vi "UHR-Fleezers Control (host) - 11.8.vi"() -> ()   [LabVIEW 2014] (continued)
        n2877 = Add(x=w4204, y=w4203) -> (x+y=w4202:dbl[][])
        n2878 = Divide(x=w4195, y=2) -> (x/y=w4193:dbl[][])
        n2879 = Divide(x=w4209, y=2) -> (x/y=w4154:dbl[][])
        n2880 = Divide(x=w4202, y=2) -> (x/y=w4156:dbl[][])
        n2881 = To Single Precision Float(number=w4189) -> (single precision float=w4188:sgl[][])
        n2882 = Transpose 2D Array(2D array=w4193) -> (transposed array=→"Data map":dbl[][])
        n2883 = To Single Precision Float(number=w4125) -> (single precision float=w4129:sgl[][])
        n2884 = To Single Precision Float(number=w4154) -> (single precision float=w4160:sgl[][])
        n2885 = To Single Precision Float(number=w4156) -> (single precision float=w4157:sgl[][])
        n2886 = call "IMAQ ArrayToImage"("Image Pixels (Float)"=w4188, "Image"=w4122) -> ("Image Out"=w4191:T2)  [unwired: 8 in, 1 out]
        n2887 = call "IMAQ ArrayToImage"("Image Pixels (Float)"=w4129, "Image"=w4121) -> ("Image Out"=w4131:T2)  [unwired: 8 in, 1 out]
        n2888 = call "IMAQ ArrayToImage"("Image Pixels (Float)"=w4160, "Image"=w4120) -> ("Image Out"=w4162:T2)  [unwired: 8 in, 1 out]
        n2889 = call "IMAQ ArrayToImage"("Image Pixels (Float)"=w4157, "Image"=w4119) -> ("Image Out"=w4159:T2)  [unwired: 8 in, 1 out]
        n2890 = call "IMAQ Symmetry"("Type of Symmetry"=w4190, "Image Src"=w4191) -> ("Image Dst Out"=w4186:T2)  [unwired: 3 in, 1 out]
        n2891 = call "IMAQ Symmetry"("Type of Symmetry"=w4130, "Image Src"=w4131) -> ("Image Dst Out"=w4127:T2)  [unwired: 3 in, 1 out]
        n2892 = call "IMAQ Symmetry"("Type of Symmetry"=w4161, "Image Src"=w4162) -> ("Image Dst Out"=→"Detection Laser X":T2)  [unwired: 3 in, 1 out]
        n2893 = call "IMAQ Symmetry"("Type of Symmetry"=w4158, "Image Src"=w4159) -> ("Image Dst Out"=→"Detection Laser Y":T2)  [unwired: 3 in, 1 out]
        n2894 = call "IMAQ Set Simple Calibration"("Calibration Axis Info"=T36 {"Origin Pixel"={"X"=0.0, "Y"=0.0}, "Angle Relative to Horizontal (deg)"=0.0, "Axis Reference"=0}, "Grid Descriptor"=T37 {"X Step"=0.3, "Y Step"=0.3, "Unit"=enum."Undefined"}, "Image"=w4186) -> ("Calibrated Image"=→"APD 1":T2)  [unwired: 7 in, 1 out]
        n2895 = call "IMAQ Set Simple Calibration"("Calibration Axis Info"=T36 {"Origin Pixel"={"X"=0.0, "Y"=0.0}, "Angle Relative to Horizontal (deg)"=0.0, "Axis Reference"=0}, "Grid Descriptor"=T37 {"X Step"=0.3, "Y Step"=0.3, "Unit"=enum."Undefined"}, "Image"=w4127) -> ("Calibrated Image"=→"APD 2":T2)  [unwired: 7 in, 1 out]
      }
    }
    n2896 = Subtract(x=w3570, y="APD 2 Offset") -> (x-y=w3567:waveform(dbl))
    n2897 = Subtract(x=w3572, y="APD 1 Offset") -> (x-y=w3568:waveform(dbl))
    n2898 = Index Array(array=w3587, index=3) -> (element=w3647:waveform(dbl))
    n2899 = Index Array(array=w3587, index=6) -> (element=w3644:waveform(dbl))
    n2900 = Build Array(w3568, w3567) -> (→"APD Chart":waveform(dbl)[])
    n2901 = Array Size(array=w3638) -> (size(s)=w3691:i32)
    n2902 = call <vilib>:"Std Deviation and Variance.vi"("X"=w3580) -> ("standard deviation"=w3579:dbl)  [unwired: 1 in, 2 out]
    n2903 = Add Array Elements(numeric array=w3580) -> (sum=w3582:u32)
    n2904 = Add Array Elements(numeric array=w3638) -> (sum=w3701:u32)
    n2905 = call <vilib>:"Std Deviation and Variance.vi"("X"=w3638) -> ("standard deviation"=w3637:dbl)  [unwired: 1 in, 2 out]
    n2906 = Divide(x="T1 offset_x (mV)", y=1000.0) -> (x/y=w3648:dbl)
    n2907 = Divide(x=w3579, y=w3578) -> (x/y=w3575:dbl)
    "Rate sigma (Hz) 2" <- w3575
    n2908 = Multiply(x=w3578, y=w3691) -> (x*y=w3581:dbl)
    "Int. Time (s)" <- w3581
    n2909 = Divide(x=w3582, y=w3581) -> (x/y=w3576:dbl)
    "APD 2 Rate (Hz)" <- w3576
    n2910 = Divide(x=w3701, y=w3581) -> (x/y=w3635:dbl)
    "APD 1 Rate (Hz)" <- w3635
    n2911 = Divide(x=w3637, y=w3578) -> (x/y=w3636:dbl)
    "Rate sigma (Hz)" <- w3636
    n2912 = Divide(x=w3575, y=w3576) -> (x/y=→"Sigma/Mean 2":dbl)
    n2913 = Divide(x=w3636, y=w3635) -> (x/y=→"s/Mean":dbl)
    n2914 = feedback-in #26("Calibration") -> ()
    n2915 = feedback #26(u16 1 ("Calibration")) -> (w3668:u16)
    n2916 = Divide(x="T2 offset_x (mV)", y=1000.0) -> (x/y=w3646:dbl)
    n2917 = case shown="0, Default" "Calibration" {
      tunnel: "T1 a_x (nm/V)" -> [_ w4085 w4106]
      tunnel: "T1 k_x (pN/nm)" -> [_ _ w4096]
      tunnel: "T2 a_x (nm/V)" -> [_ w4084 w4104]
      tunnel: "T2 k_x (pN/nm)" -> [_ _ w4097]
      tunnel: w3647 -> [w4067 w4082 w4102]
      tunnel: w3644 -> [w4066 w4080 w4100]
      tunnel: [w4067 w4079 w4099] -> w3677
      tunnel: [w4066 w4078 w4098] -> w3676
      tunnel: ["T1 X (V)" ("Label.Text") "T1 X (nm)" ("Label.Text") "T1 X (pN)" ("Label.Text")] -> w3665
      tunnel: ["T2 X (V)" ("Label.Text") "T2 X (nm)" ("Label.Text") "T2 X (pN)" ("Label.Text")] -> w3664
      tunnel: ["Position (V)" ("Label.Text") "Position (nm)" ("Label.Text") "Force (pN)" ("Label.Text")] -> w3666
      tunnel: w3646 -> [_ w4070 w4089]
      tunnel: w3648 -> [_ w4073 w4091]
      tunnel: ["Mean (V)" ("Label.Text") "Mean (nm)" ("Label.Text") "Mean (pN)" ("Label.Text")] -> w3661
      tunnel: ["Difference (V)" ("Label.Text") "Difference (nm)" ("Label.Text") "Difference (pN)" ("Label.Text")] -> w3595
      frame 0, Default {
      }
      frame 1 {
        n2918 = Unbundle By Name(w4082) -> ("Y"=w4086:dbl[])
        n2919 = Unbundle By Name(w4080) -> ("Y"=w4071:dbl[])
        n2920 = Subtract(x=w4086, y=w4073) -> (x-y=w4074:dbl[])
        n2921 = Subtract(x=w4071, y=w4070) -> (x-y=w4072:dbl[])
        n2922 = Multiply(x=w4072, y=w4084) -> (x*y=w4081:dbl[])
        n2923 = Multiply(x=w4085, y=w4074) -> (x*y=w4083:dbl[])
        n2924 = Bundle By Name(cluster=w4080, "Y"=w4081) -> (w4078:waveform(dbl))
        n2925 = Bundle By Name(cluster=w4082, "Y"=w4083) -> (w4079:waveform(dbl))
      }
      frame 2 {
        n2926 = Unbundle By Name(w4102) -> ("Y"=w4107:dbl[])
        n2927 = Unbundle By Name(w4100) -> ("Y"=w4105:dbl[])
        n2928 = Subtract(x=w4105, y=w4089) -> (x-y=w4090:dbl[])
        n2929 = Subtract(x=w4107, y=w4091) -> (x-y=w4092:dbl[])
        n2930 = Compound Arithmetic op=MULTIPLY(w4090, w4104, w4097) -> (w4101:dbl[])
        n2931 = Compound Arithmetic op=MULTIPLY(w4096, w4106, w4092) -> (w4103:dbl[])
        n2932 = Bundle By Name(cluster=w4100, "Y"=w4101) -> (w4098:waveform(dbl))
        n2933 = Bundle By Name(cluster=w4102, "Y"=w4103) -> (w4099:waveform(dbl))
      }
    }
    n2934 = Not Equal?(x=w3668, y="Calibration") -> (x != y?=w3625:bool)
    n2935 = case shown="True" w3625 {
      tunnel: w3666 -> [_ w4060]
      tunnel: w3665 -> [_ w4059]
      tunnel: w3664 -> [_ w4058]
      tunnel: w3661 -> [_ w4057]
      tunnel: w3595 -> [_ w4056]
      frame False {
      }
      frame True {
        n2936 = property on="Force" class="WFChart (strict)"("YScale.NameLbl.Text"=w4060) -> ()  [unwired: 2 in, 2 out]
        n2937 = property on="T2 X" class="DigNum (strict)"("Caption.Text"=w4058) -> ()  [unwired: 2 in, 2 out]
        n2938 = property on="T1 X" class="DigNum (strict)"("Caption.Text"=w4059) -> ()  [unwired: 2 in, 2 out]
        n2939 = property on="Mean" class="DigNum (strict)"("Caption.Text"=w4057) -> ()  [unwired: 2 in, 2 out]
        n2940 = property on="Difference" class="DigNum (strict)"("Caption.Text"=w4056) -> ()  [unwired: 2 in, 2 out]
      }
    }
    n2941 = Unbundle By Name(w3647) -> ("Y"=w3650:dbl[])
    n2942 = Unbundle By Name(w3644) -> ("Y"=w3653:dbl[])
    n2943 = Subtract(x=w3650, y=w3648) -> (x-y=w3651:dbl[])
    n2944 = Subtract(x=w3653, y=w3646) -> (x-y=w3652:dbl[])
    n2945 = Multiply(x=w3652, y="T2 a_x (nm/V)") -> (x*y=w3440:dbl[])
    n2946 = Multiply(x="T1 a_x (nm/V)", y=w3651) -> (x*y=w3441:dbl[])
    n2947 = Not(x="Trap Trig. Fl.") -> (.not. x?=w3477:bool)
    n2948 = Multiply(x=w3676, y=-1.0) -> (x*y=w3655:waveform(dbl))
    n2949 = Subtract(x=w3441, y=w3440) -> (x-y=w3643:dbl[])
    n2950 = Unbundle By Name(w3676) -> ("Y"=w3614:dbl[])
    n2951 = Unbundle By Name(w3677) -> ("Y"=w3442:dbl[])
    n2952 = Negate(x=w3643) -> (-x=w3438:dbl[])
    n2953 = Build Array(w3677, w3655) -> (→"Force":waveform(dbl)[])
    n2954 = Subtract(x=w3438, y="Offset (nm)") -> (x-y=w3612:dbl[])
    n2955 = case shown="True" "Read Lateness and Rel Phase" {
      tunnel: w3458 -> [w4033 w4055]
      tunnel: w3457 -> [w4034 w4054]
      tunnel: [w4033 w4053] -> w3641
      tunnel: [w4034 w4052] -> w3640
      frame False {
      }
      frame True {
        n2956 = xnode "Read/Write Control"("FPGA VI Reference In"=w4055, "error in"=w4054) -> ("FPGA VI Reference Out"=w4053:T19, "error out"=w4052:errorcluster, "GI Relative phase"=→"GI relative phase":i16, "Relative phase"=→"Relative phase (AI1)":i16, "AI Late Counter"=→"Late Counter (AI1)":u8, "GI Late Counter"=→"GI Late Counter":u8, "MCL Late Counter"=→"MCL Late Counter":u8, "MCL Relative Phase"=→"Relative Phase (MCL)":i16, "APD Acq Relative Phase"=→"APD Acq Relative Phase":i16, "APD 1 Gate Relative Phase"=→"APD 1 Gate Relative Phase":i16, "APD 2 Gate Relative Phase"=→"APD 2 Gate Relative Phase":i16, "APD Acq Late Counter"=→"APD Acq Late Counter":u8, "APD 1 Gate Late Counter"=→"APD 1 Gate Late Counter":u8, "APD 2 Gate Late Counter"=→"APD 2 Gate Late Counter":u8, "Green FB Relative Phase"=→"Relative phase (Green FB)":i16, "GI Relative phase 2"=→"GI relative phase 2":i16, "GI Late Counter 2"=→"GI Late Counter 2":u8, "Trap Pos FIFO Timeout"=→"Trap Pos FIFO Timeout":u16, "Trap AI FIFO Timeout"=→"Trap AI FIFO Timeout":u16)
      }
    }
    n2957 = call-poly <vilib>:"Mean.vi"("X"=w3614) -> ("mean"=w3444:dbl)  [unwired: 1 out]
    "T2 X" <- w3444
    n2958 = Negate(x=w3614) -> (-x=w3615:dbl[])
    n2959 = call-poly <vilib>:"Mean.vi"("X"=w3442) -> ("mean"=w3445:dbl)  [unwired: 1 out]
    "T1 X" <- w3445
    n2960 = Negate(x=w3444) -> (-x=w3443:dbl)
    n2961 = Bundle By Name(cluster=w3647, "Y"=w3612) -> (w3586:waveform(dbl))
    "Bead Separation" <- w3586
    n2962 = Add(x=w3442, y=w3615) -> (x+y=w3616:dbl[])
    n2963 = Add(x=w3445, y=w3443) -> (x+y=w3663:dbl)
    n2964 = Subtract(x=w3445, y=w3443) -> (x-y=→"Difference":dbl)
    n2965 = Divide(x=w3616, y=2.0) -> (x/y=→"Vec Mean of T1 T2":dbl[])
    n2966 = Divide(x=w3663, y=2.0) -> (x/y=w3618:dbl)
    "Mean" <- w3618
    n2967 = feedback-in #27("Trap Trig. Fl.") -> ()
    n2968 = feedback #27("Trap Trig. Fl.") -> (w3475:bool)
    n2969 = And(x=w3477, y=w3475) -> (x .and. y?=w3476:bool)
    n2970 = case "If have just turned off triggering" shown="True" w3476 {
      tunnel: w3458 -> [_ w3863]
      tunnel: w3457 -> [_ w3862]
      frame False {
      }
      frame True {
        w3861 = FALSE ("FPGA Trap Trig")
        n2971 = xnode "Read/Write Control"("FPGA VI Reference In"=w3863, "error in"=w3862, "FPGA Trap Trig"=w3861) -> ("FPGA VI Reference Out"=w3860:T19, "error out"=w3859:errorcluster)
        n2972 = xnode "Read/Write Control"("FPGA VI Reference In"=w3860, "error in"=w3859, "TTrig?"=w3861) -> ()  [unwired: 2 out]
        n2973 = local write "Initializing"(FALSE ("Initializing")) -> ()
        n2974 = local write "Triggered"(FALSE ("Triggered")) -> ()
        n2975 = local write "Waiting"(FALSE ("Waiting")) -> ()
      }
    }
    n2976 = Not(x=w3475) -> (.not. x?=w3488:bool)
    n2977 = And(x="Trap Trig. Fl.", y=w3488) -> (x .and. y?=w3485:bool)
    n2978 = local read "Tether"() -> (w3619:bool)
    n2979 = Or(x=w3485, y="Reinitialize") -> (x .or. y?=w3471:bool)
    n2980 = feedback #28(w3481) -> (w3486:string)
    n2981 = Select(t=w3481, s=w3485, f=w3486) -> (s? t:f=w3480:string)
    n2982 = Select(t=w3481, s="Reinitialize", f=w3480) -> (s? t:f=w3479:string)
    n2983 = feedback #29(0) -> (w3483:i32)
    n2984 = feedback #30(w3612) -> (w3611:dbl[])
    n2985 = Build Array (concatenate)(w3612, w3611) -> (w3439:dbl[])
    n2986 = case "For determining if there is a tether still" shown="True" w3619 {
      tunnel: w3618 -> [_ w3987]
      frame False {
      }
      frame True {
        n2987 = Greater?(x="Lost Tether Alarm Threshold (pN)", y=w3987) -> (0:w3985:bool)
        n2988 = case shown="True" w3985 {
          frame False {
          }
          frame True {
            w3988 = TRUE
            w3992 = FALSE ("Multiple tether")
            w3993 = FALSE ("Value (Signaling)")
            n2989 = flat-sequence {
              frame #0 {
                # "stop only if saving"
                n2990 = local read "Saving..."() -> (w4005:bool)
                n2991 = And(x=w4005, y="TA Cancel Save?") -> (x .and. y?=w4004:bool)
                n2992 = local write "Stop Saving"(w4004) -> ()
              }
              frame #1 {
                n2993 = case shown="True" "TA Green Off?" {
                  frame False {
                  }
                  frame True {
                    w4008 = FALSE ("Fl. Triggered...")
                    n2994 = local write "Fl. Triggered..."(w4008) -> ()
                    n2995 = property on="Green Laser ON/Interlacing" class="Bool (strict)"("Val(Sgnl)"=w4008) -> ()  [unwired: 2 in, 2 out]
                  }
                }
              }
            }
            n2996 = local read "Time tether formed"() -> (w3999:timestamp)
            n2997 = Get Date/Time In Seconds() -> (seconds since 1Jan1904=w4000:timestamp)
            n2998 = Subtract(x=w4000, y=w3999) -> (x-y=w3998:dbl)
            n2999 = Number To Decimal String(number=w3998) -> (decimal integer string=w3995:string)  [unwired: 1 out]
            n3000 = local read "Messages"() -> (w4002:string)
            n3001 = call <vilib>:"Beep.vi"("use system alert? (T)"=FALSE, "duration (msec)"=u32 200, "frequency (Hz)"=u32 200) -> ()  [unwired: 9 out]
            n3002 = Concatenate Strings("Lost tether (" ("Message to add"), w3995, " s)." ("string")) -> (w3997:string)
            n3003 = local write "Tether"(FALSE ("Tether")) -> ()
            n3004 = call "Update messages.vi"("Message to add"=w3997, "Old message string"=w4002) -> ("New message string"=w4001:string)
            n3005 = local write "Messages"(w4001) -> ()
            n3006 = local write "Pause dwell"(w3993) -> ()
            n3007 = property on="Fl. Triggered..." class="Bool (strict)"("Val(Sgnl)"=w3993) -> ()  [unwired: 2 in, 2 out]
            n3008 = local write "Dip for Protein"(w3993) -> ()
            n3009 = property on="Trap Pos. FB ON" class="Bool (strict)"("Val(Sgnl)"=w3993) -> ()  [unwired: 2 in, 2 out]
            n3010 = property on="Trap Trig. Fl." class="Bool (strict)"("Val(Sgnl)"=w3993) -> ()  [unwired: 2 in, 2 out]
            n3011 = local write "Multiple tether"(w3992) -> ()
            n3012 = local write "Bad fit"(w3992) -> ()
            n3013 = local write "Hysteresis"(w3992) -> ()
            n3014 = local write "Good tether"(w3992) -> ()
            n3015 = local write "Save scans"(w3988) -> ()
            n3016 = local write "Restart DMA? (AOD)"(w3988) -> ()
          }
        }
      }
    }
    n3017 = case "For triggering actions based on the trap position (e.g., turning the excitation laser on if trap under feedback moves so far)" shown="True" "Trap Trig. Fl." {
      tunnel: w3466 -> [_ w3876]
      tunnel: w3479 -> [_ w3875]
      tunnel: ["" ("t") w3874] -> w3487
      tunnel: w3471 -> [_ w3873]
      tunnel: [0 ("t") w3872] -> w3484
      tunnel: w3483 -> [_ w3871]
      tunnel: w3458 -> [_ w3870]
      tunnel: w3457 -> [_ w3869]
      frame False {
      }
      frame True {
        n3018 = case shown="\"Wait for trigger\"" w3875 {
          tunnel: w3876 -> [w3893 _ _ w3941]
          tunnel: [w3890 w3922 "" ("t") w3944] -> w3874
          tunnel: w3873 -> [_ _ _ w3932]
          tunnel: [w3889 w3919 0 ("t") w3933] -> w3872
          tunnel: w3871 -> [_ w3921 _ w3939]
          tunnel: w3870 -> [w3878 w3916 _ w3935]
          tunnel: w3869 -> [w3877 w3915 _ w3934]
          frame "Wait for trigger" {
            n3019 = local read "Trap Trig. (FPGA)"() -> (w3881:bool)
            n3020 = Subtract(x=w3893, y="Mean T1 Position\nto compare (nm)") -> (x-y=w3886:dbl[])
            n3021 = call <vilib>:"Std Deviation and Variance.vi"("X"=w3886) -> ("mean"=→"mean":dbl, "standard deviation"=→"standard\ndeviation":dbl)  [unwired: 1 in, 1 out]
            n3022 = Array Max & Min(array=w3886) -> (max value=→"max value":dbl, min value=→"min value":dbl)  [unwired: 2 out]
            n3023 = Greater?(x=w3886, y="Threshold (nm)") -> (0:w3896:bool[])
            n3024 = case shown="True" w3881 {
              tunnel: w3878 -> [_ w3902]
              tunnel: w3877 -> [_ w3901]
              tunnel: [FALSE ("TTrig?") w3900] -> w3884
              frame False {
              }
              frame True {
                n3025 = xnode "Read/Write Control"("FPGA VI Reference In"=w3902, "error in"=w3901) -> ("TTrig?"=w3900:bool)  [unwired: 2 out]
              }
            }
            n3026 = Or Array Elements(Boolean array=w3896) -> (logical OR=w3883:bool)
            n3027 = Select(t=w3884, s=w3881, f=w3883) -> (s? t:f=w3882:bool)
            n3028 = Not(x=w3881) -> (.not. x?=w3880:bool)
            n3029 = And(x=w3882, y=w3880) -> (x .and. y?=w3879:bool)
            n3030 = Select(t="Triggered", s=w3882, f="Wait for trigger") -> (s? t:f=w3890:string)
            n3031 = case shown="True" w3882 {
              tunnel: [0 0] -> w3889
              tunnel: w3878 -> [_ w3907]
              tunnel: w3877 -> [_ w3906]
              frame False {
                "Waiting" <- TRUE ("Waiting")
              }
              frame True {
                n3032 = xnode "Read/Write Control"("FPGA VI Reference In"=w3907, "error in"=w3906, "TTrig?"=FALSE) -> ()  [unwired: 2 out]
                n3033 = local read "Messages"() -> (w3910:string)
                n3034 = call <vilib>:"Beep.vi"() -> ()  [unwired: 12 in]
                n3035 = call "Update messages.vi"("Message to add"="Unwinding trigger.", "Old message string"=w3910) -> ("New message string"=w3911:string)
                n3036 = local write "Messages"(w3911) -> ()
                n3037 = local write "Waiting"(FALSE ("Waiting")) -> ()
                "Triggered" <- TRUE ("Triggered")
              }
            }
            n3038 = case "Only need to turn on laser if host triggered" shown="True" w3879 {
              frame False {
              }
              frame True {
                n3039 = property on="Green Laser ON/Interlacing" class="Bool (strict)"("Val(Sgnl)"=TRUE ("Value (Signaling)")) -> ()  [unwired: 2 in, 2 out]
              }
            }
          }
          frame "Triggered" {
            n3040 = local read "Trap Trig. (FPGA)"() -> (w3918:bool)
            n3041 = Increment(x=w3921) -> (x+1=w3919:i32)
            n3042 = Greater Or Equal?(x=w3919, y="Fl. ON time (n)") -> (x >= y?=w3917:bool)
            n3043 = Select(t="Wait for trigger", s=w3917, f="Triggered" ("t")) -> (s? t:f=w3922:string)
            n3044 = And(x=w3917, y=w3918) -> (x .and. y?=w3914:bool)
            n3045 = case shown="True" w3914 {
              tunnel: w3916 -> [_ w3926]
              tunnel: w3915 -> [_ w3925]
              frame False {
              }
              frame True {
                n3046 = xnode "Read/Write Control"("FPGA VI Reference In"=w3926, "error in"=w3925, "FPGA Trap Trig"=TRUE) -> ()  [unwired: 2 out]
              }
            }
            n3047 = case shown="True" w3917 {
              frame False {
              }
              frame True {
                w3928 = FALSE ("Value (Signaling)")
                n3048 = local write "Triggered"(w3928) -> ()
                n3049 = local write "Waiting"(TRUE ("Waiting")) -> ()
                n3050 = property on="Green Laser ON/Interlacing" class="Bool (strict)"("Val(Sgnl)"=w3928) -> ()  [unwired: 2 in, 2 out]
              }
            }
          }
          frame "Do nothing" {
          }
          frame "Initialize", Default {
            n3051 = Increment(x=w3939) -> (x+1=w3943:i32)
            n3052 = Select(t=1, s=w3932, f=w3943) -> (s? t:f=w3933:i32)
            n3053 = feedback #31(w3941) -> (w3947:dbl[])
            n3054 = Build Array (concatenate)(w3941, w3947) -> (w3940:dbl[])
            n3055 = Greater Or Equal?(x=w3933, y="Wait to get offset (n)") -> (x >= y?=w3936:bool)
            n3056 = Select(t=w3941, s=w3932, f=w3940) -> (s? t:f=w3942:dbl[])
            n3057 = feedback-in #31(w3942) -> ()
            n3058 = call-poly <vilib>:"Mean.vi"("X"=w3942) -> ("mean"=w3937:dbl)  [unwired: 1 out]
            n3059 = local write "Mean T1 Position\nto compare (nm)"(w3937) -> ()
            n3060 = case shown="True" w3932 {
              tunnel: w3935 -> [_ w3953]
              tunnel: w3934 -> [_ w3952]
              frame False {
              }
              frame True {
                w3949 = FALSE ("FPGA Trap Trig")
                n3061 = xnode "Read/Write Control"("FPGA VI Reference In"=w3953, "error in"=w3952, "FPGA Trap Trig"=w3949) -> ("FPGA VI Reference Out"=w3951:T19, "error out"=w3950:errorcluster)
                n3062 = xnode "Read/Write Control"("FPGA VI Reference In"=w3951, "error in"=w3950, "TTrig?"=w3949) -> ()  [unwired: 2 out]
              }
            }
            n3063 = Select(t="Wait for trigger", s=w3936, f="Initialize") -> (s? t:f=w3944:string)
            n3064 = case shown="True" w3936 {
              tunnel: w3937 -> [_ w3956]
              tunnel: w3935 -> [_ w3965]
              tunnel: w3934 -> [_ w3964]
              frame False {
                n3065 = local write "Waiting"(FALSE ("Waiting")) -> ()
                "Initializing" <- TRUE ("Initializing")
              }
              frame True {
                n3066 = local read "Threshold (nm)"() -> (w3968:dbl)
                n3067 = local read "AOM X Cal (nm/MHz)"() -> (w3967:dbl)
                n3068 = Add(x=w3956, y=w3968) -> (x+y=w3969:dbl)
                n3069 = Divide(x=w3969, y=w3967) -> (x/y=w3966:dbl)
                n3070 = call "IR AOM freq to word.vi"("Frequency In (MHz)"=w3966) -> ("Frequency Word Out (double)"=w3963:dbl)
                n3071 = local write "Initializing"(FALSE ("Initializing")) -> ()
                n3072 = local write "Waiting"(TRUE ("Waiting")) -> ()
                n3073 = To Quad Integer(1:w3963) -> (0:w3962:i64)
                n3074 = xnode "Read/Write Control"("FPGA VI Reference In"=w3965, "error in"=w3964, "FPGA TTrig Thresh"=w3962) -> ("FPGA VI Reference Out"=w3959:T19, "error out"=w3958:errorcluster)
                n3075 = xnode "Read/Write Control"("FPGA VI Reference In"=w3959, "error in"=w3958, "FPGA Trap Trig"=TRUE) -> ()  [unwired: 2 out]
              }
            }
          }
        }
      }
    }
    n3076 = feedback-in #28(w3487) -> ()
    n3077 = feedback-in #29(w3484) -> ()
    n3078 = Split 1D Array(array=w3439, index=w3501) -> (first subarray=w3608:dbl[])  [unwired: 1 out]
    n3079 = feedback-in #30(w3608) -> ()
    n3080 = call-poly <vilib>:"Mean.vi"("X"=w3608) -> ("mean"=w3607:dbl)  [unwired: 1 out]
    "Bead Mean (nm)" <- w3607
    n3081 = Subtract(x=w3608, y=w3607) -> (x-y=w3606:dbl[])
    n3082 = Square(x=w3606) -> (x^2=w3605:dbl[])
    n3083 = call-poly <vilib>:"Mean.vi"("X"=w3605) -> ("mean"=w3604:dbl)  [unwired: 1 out]
    n3084 = Square Root(x=w3604) -> (sqrt(x)=w3603:dbl)
    n3085 = Multiply(x=10.0, y=w3603) -> (x*y=→"RMS (Å)":dbl)
    n3086 = xnode ("Read/Write Control")("FPGA VI Reference In"=w3641, "error in"=w3640) -> ("FPGA VI Reference Out"=w3469:T19, "error out"=w3468:errorcluster, "AI2 Y Sum Set 1"=w3746:i16, "AI2 Y Sum Set 2"=w3745:i16, "AI1 X Set 1"=w3532:fxp<+/-,16,1>, "AI1 X Set 2"=w3531:fxp<+/-,16,1>, "Trap Pos FB Int Signal"=→"Trap Pos FB Int Signal":fxp<+/-,24,9>, "Trap Pos FB Int-Norm Signal"=→"Trap Pos FB Int-Norm Signal":fxp<+/-,16,1>, "Trap Pos FB Action"=w3525:i64, "Scanning"=→"AOD Scanning":bool, "Scan I"=→"AOD Scan I":u64, "Scanning MCL"=w3748:bool, "Scan I (MCL)"=→"MCL Scan I":u64, "Green FB Signals"=w3686:T47, "Trap Pos FB Action"=w3456:i64, "Wiggling 1"=→"Wiggling T1":bool, "TTrig Fin Thresh"=w3452:i64, "Wiggling 2"=→"Wiggling T2":bool)  [unwired: 2 out]
    "MCL Scanning" <- w3748
    "Trap Pos FB Action" <- w3525
    n3087 = local read "FB Trig Integrate"() -> (w3450:u32)
    n3088 = Divide(x=w3456, y=w3450) -> (x/y=w3449:dbl)
    "TTrig Sig (Int)" <- w3449
    n3089 = Divide(x=w3452, y=w3450) -> (x/y=w3447:dbl)
    "TTrig Fin Thresh (Int)" <- w3447
    n3090 = local read "AOM X Cal (nm/MHz)"() -> (w3455:dbl)
    n3091 = local read "AI2 (V)"() -> (w3747:cluster{"Set 1":dbl, "Set 2":dbl})
    n3092 = Bundle By Name(cluster=w3747, "Set 1"=w3746, "Set 2"=w3745) -> (w3743:cluster{"Set 1":dbl, "Set 2":dbl})
    n3093 = Divide(x=w3525, y=327.67) -> (x/y=w3434:dbl)
    n3094 = local read "Trap X (AI1)"() -> (w3545:T10)
    n3095 = call "IR AOM word double to freq.vi"("Frequency Word In (double)"=w3447) -> ("Frequency Out (MHz)"=w3446:dbl)
    n3096 = call "IR AOM word double to freq.vi"("Frequency Word In (double)"=w3449) -> ("Frequency Out (MHz)"=w3448:dbl)
    n3097 = Divide(x=w3743, y=3276.7) -> (x/y=w3742:cluster{"Set 1":dbl, "Set 2":dbl})
    n3098 = Multiply(x=w3448, y=w3455) -> (x*y=w3454:dbl)
    "TTrig Sig (nm)" <- w3454
    n3099 = Multiply(x=w3446, y=w3455) -> (x*y=w3453:dbl)
    "TTrig Fin Thresh (nm)" <- w3453
    n3100 = local write "AI2 (V)"(w3742) -> ()
    n3101 = local read "Trap Pos. FB Range"() -> (w3433:T12)
    n3102 = Bundle(cluster=w3545, "Trap 1"=w3532, "Trap 2"=w3531) -> (→"Trap X (AI1)":T10)
    n3103 = Bundle(w3454, w3453) -> (→"TTrig":cluster{dbl, dbl})  [unwired: 1 in]
    n3104 = Unbundle(w3433) -> ("output high"=w3432:fxp<+/-,64,32>)  [unwired: 1 out]
    n3105 = Divide(x=w3434, y=w3432) -> (x/y=→"Action (%)":dbl)
    n3106 = Divide(x=w3686, y=3276.7) -> (x/y=w3682:T48)
    n3107 = Unbundle By Name(w3682) -> ("Green FB Ch 0"=w3685:dbl, "Green FB Ch 1"=w3684:dbl, "Green FB Ch 2"=w3683:dbl)
    n3108 = Divide(x=w3685, y=w3683) -> (x/y=w3681:dbl)
    n3109 = Divide(x=w3684, y=w3683) -> (x/y=w3680:dbl)
    n3110 = flat-sequence "To save data" {
      tunnel: [w4829] -> w3766
      tunnel: [w4830] -> w3765
      tunnel: w3717 -> [w4802]
      tunnel: w3474 -> [w4827]
      tunnel: ["Save Calibration"] -> w3739
      tunnel: w3736 -> [w4826]
      tunnel: [w4820] -> w3735
      tunnel: [w4817] -> w3734
      tunnel: [w4814] -> w3733
      tunnel: w3716 -> [w4816]
      tunnel: w3623 -> [w4810]
      tunnel: [w4810] -> w3622
      tunnel: ["Start Saving"] -> w3588
      tunnel: [w4804] -> w3514
      tunnel: [w4803] -> w3513
      tunnel: w3766 -> [w5069]
      tunnel: w3765 -> [w5068]
      tunnel: w3515 -> [w5067]
      tunnel: w3739 -> [w5066]
      tunnel: w3735 -> [w5064]
      tunnel: w3734 -> [w5063]
      tunnel: w3733 -> [w5062]
      tunnel: w3597 -> [w5061]
      tunnel: w3633 -> [w5060]
      tunnel: w3622 -> [w5059]
      tunnel: w3588 -> [w5058]
      tunnel: w3586 -> [w5057]
      tunnel: w3562 -> [w5056]
      tunnel: w3514 -> [w5055]
      tunnel: w3513 -> [w5054]
      tunnel: w3512 -> [w5053]
      tunnel: w3435 -> [w5052]
      frame #0 {
        n3111 = Or(x="Save N Sets", y="Start Saving") -> (x .or. y?=w4811:bool)
        n3112 = To Double Precision Float(number=w4826) -> (double precision float=w4821:dbl)
        n3113 = Build Array(w4811, "Save Calibration", w4802, w4816) -> (w4825:bool[])
        n3114 = Compound Arithmetic op=OR("Save Calibration", w4802, w4811, w4816) -> (w4828:bool)
        n3115 = Boolean Array To Number(Boolean array=w4825) -> (number=w4823:u32)
        n3116 = feedback #32(FALSE ("Save APD Data\nwith Trap Data")) -> (w4805:bool)
        n3117 = feedback #33(refnum<k0> refnum) -> (w4831:refnum<file>)
        n3118 = feedback #34(refnum<k0> refnum) -> (w4807:refnum<file>)
        n3119 = feedback #35(FALSE ("Save APD Data\nwith Trap Data")) -> (w4815:bool)
        n3120 = feedback #36(refnum<k0> refnum) -> (w4818:refnum<file>)
        n3121 = feedback #37(0) -> (w4833:i32)
        n3122 = feedback #38() -> (w4822:u32)  [unwired: 1 out]
        n3123 = case shown="True" w4828 {
          tunnel: [w4840 1] -> w4829
          tunnel: w4833 -> [w4842 _]
          tunnel: [w4841 w4860] -> w4830
          tunnel: w4831 -> [w4841 _]
          tunnel: w4827 -> [_ w4880]
          tunnel: w4821 -> [_ w4878]
          tunnel: w4823 -> [_ w4881]
          tunnel: [w4839 w4859] -> w4820
          tunnel: w4822 -> [w4839 _]
          tunnel: [w4838 w4857] -> w4817
          tunnel: w4818 -> [w4838 _]
          tunnel: [w4837 w4856] -> w4814
          tunnel: w4815 -> [w4837 _]
          tunnel: "Start Saving" -> [_ w4854]
          tunnel: w4810 -> [_ w4853]
          tunnel: [w4836 w4844] -> w4803
          tunnel: w4807 -> [w4836 _]
          tunnel: [w4835 w4843] -> w4804
          tunnel: w4805 -> [w4835 _]
          frame False {
            n3124 = Increment(x=w4842) -> (x+1=w4840:i32)
          }
          frame True {
            w4850 = FALSE ("Start Saving")
            w4855 = 9.0  # File Version
            w4863 = FALSE ("prepend array or string size? (T)")
            w4861 = T24."big-endian, network order" ("byte order (0:big-endian, network order)")
            n3125 = local read "BD 1 Frequency 1 (MHz)"() -> (w4877:dbl)
            n3126 = local read "BD 2 Frequency 1 (MHz)"() -> (w4876:dbl)
            n3127 = local read "BD 1 Frequency 2 (MHz)"() -> (w4875:dbl)
            n3128 = local read "BD 2 Frequency 2 (MHz)"() -> (w4874:dbl)
            n3129 = local read "BD 1 Frequency 3 (MHz)"() -> (w4873:dbl)
            n3130 = local read "BD 2 Frequency 3 (MHz)"() -> (w4872:dbl)
            n3131 = Array Size(array=w4853) -> (size(s)=w4852:i32)
            n3132 = To Double Precision Float(number=w4852) -> (double precision float=w4851:dbl)
            n3133 = local write "Save Calibration"(w4850) -> ()
            n3134 = local write "Start Saving"(w4850) -> ()
            n3135 = Build Array("Save APD Data\nwith Trap Data", "Save Trap Pos. Data") -> (w4847:bool[])
            n3136 = Boolean Array To Number(Boolean array=w4847) -> (number=w4846:u32)
            n3137 = Build Array(w4877, w4876, w4875, w4874, w4873, w4872) -> (w4871:dbl[])
            n3138 = case shown="1, Default" w4881 {
              tunnel: w4880 -> [w4954 w4976 w4992 w5030]
              tunnel: w4851 -> [w4959 w4983 w5012 w5049]
              tunnel: w4878 -> [w4958 w4982 w5011 w5048]
              tunnel: [w4955 w4978 w5003 w5040] -> w4869
              tunnel: [w4947 "Cal sets to save" w4993 w5031] -> w4859
              tunnel: w4871 -> [w4956 w4979 w5005 w5042]
              tunnel: "Save APD Data\nwith Trap Data" -> [w4953 _ w4989 w5028]
              tunnel: [w4953 FALSE ("Save APD Data\nwith Trap Data") w4989 w5028] -> w4856
              tunnel: w4855 -> [w4950 w4973 w4987 w5026]
              tunnel: w4854 -> [w4949 _ _ _]
              tunnel: [w4941 "Active cal?" w4986 w5016] -> w4843
              tunnel: "Save Trap Pos. Data" -> [w4941 _ w4986 w5016]
              tunnel: w4846 -> [w4940 _ w4985 w5015]
              frame 1, Default {
                # "timeseries"
                n3139 = case shown="True" "Profile" {
                  tunnel: [w4962 w4966] -> w4945
                  tunnel: [w4962 w4965] -> w4944
                  tunnel: [w4962 w4964] -> w4943
                  tunnel: [w4962 w4963] -> w4942
                  frame False {
                    w4962 = 0.0 ("f")
                  }
                  frame True {
                    n3140 = local read "Current Position"() -> (w4967:cluster{dbl, dbl, dbl})
                    n3141 = local read "Y change (mm)"() -> (w4963:dbl)
                    n3142 = Unbundle(w4967) -> (w4966:dbl, w4965:dbl, w4964:dbl)
                  }
                }
                n3143 = local read "Save ave N"() -> (w4961:dbl)
                n3144 = Multiply(x=w4961, y=w4954) -> (x*y=w4960:dbl)
                n3145 = To Double Precision Float(number=w4940) -> (double precision float=w4952:dbl)
                n3146 = Select(t=4.0, s="Profile", f=0.0) -> (s? t:f=w4936:dbl)
                n3147 = Build Array(w4950, w4954, w4960, w4959, w4958, w4936) -> (w4957:dbl[])
                n3148 = Build Array(w4952, w4945, w4944, w4943, w4942) -> (w4951:dbl[])
                n3149 = Select(t=u32 4000000000, s=w4949, f="N sets to save") -> (s? t:f=w4947:u32)
                n3150 = Build Array (concatenate)(w4957, w4956, w4951) -> (w4955:dbl[])
              }
              frame 2 {
                w4975 = 0.0 ("f")
                # "If doing active calibration,\nalso save trap position file"
                # "calibration"
                n3151 = property on="Wiggle" class="Bool (strict)"("Val(Sgnl)"="Active cal?") -> ()  [unwired: 2 in, 2 out]
                n3152 = Select(t=2.0, s="Active cal?", f=0.0) -> (s? t:f=w4969:dbl)
                n3153 = Build Array(w4969, w4975, w4975, w4975, w4975) -> (w4974:dbl[])
                n3154 = Build Array(w4973, w4976, w4976, w4983, w4982, 1.0 ("t")) -> (w4980:dbl[])
                n3155 = Build Array (concatenate)(w4980, w4979, w4974) -> (w4978:dbl[])
                "Calibrating..." <- TRUE ("Calibrating...")
              }
              frame 4 {
                w4990 = 0.0 ("f")
                # "scan dir (x/y = 0/1)"
                # "cycles/step"
                # "n scans (f/b)"
                # "steps"
                # "freq. range"
                # "AOD raster scan"
                n3156 = local read "Number of F/B Scans (AOD)"() -> (w4997:u16)
                n3157 = local read "Cycles/step (AOD)"() -> (w4999:u64)
                n3158 = local read "Scan Range (MHz)"() -> (w5002:dbl)
                n3159 = local read "Scan steps (AOD)"() -> (w5001:u64)
                n3160 = local read "Scan BD"() -> (w5009:bool)
                n3161 = local read "Save ave N"() -> (w5014:dbl)
                n3162 = Boolean To (0,1)(Boolean=w5009) -> (0, 1=w5008:i16)
                n3163 = To Double Precision Float(number=w4997) -> (double precision float=w4996:dbl)
                n3164 = To Double Precision Float(number=w5001) -> (double precision float=w5000:dbl)
                n3165 = To Double Precision Float(number=w4999) -> (double precision float=w4998:dbl)
                n3166 = To Double Precision Float(number=w5008) -> (double precision float=w5007:dbl)
                n3167 = Multiply(x=w5014, y=w4992) -> (x*y=w5013:dbl)
                n3168 = To Double Precision Float(number=w4985) -> (double precision float=w4991:dbl)
                n3169 = Build Array(w4991, w4990, w4990, w4990, w4990) -> (w4988:dbl[])
                n3170 = local read "N sets should be saved"() -> (w4994:dbl)
                n3171 = Build Array(w5007, w5002, w5000, w4998, w4996) -> (w5004:dbl[])
                n3172 = Build Array(w4987, w4992, w5013, w5012, w5011, 2.0 ("t")) -> (w5006:dbl[])
                n3173 = Round Toward +Infinity(x=w4994) -> (ceil(x): smallest int >= x=w4995:dbl)
                n3174 = Build Array (concatenate)(w5006, w5005, w4988, w5004) -> (w5003:dbl[])
                n3175 = To Unsigned Long Integer(number=w4995) -> (unsigned 32bit integer=w4993:u32)
              }
              frame 8 {
                w5023 = 0.0 ("f")
                # "MCL raster scan"
                n3176 = local read "Number of scans (MCL)"() -> (w5018:u64)
                n3177 = local read "Scan lines (y)"() -> (w5017:u64)
                n3178 = local read "2D or 1D Scan"() -> (w5020:bool)
                n3179 = local read "Scan Range (V)\n(of steps)"() -> (w5039:dbl)
                n3180 = local read "Fast Scan Dir"() -> (w5046:bool)
                n3181 = local read "Cycles/step (MCL)"() -> (w5036:u64)
                n3182 = local read "Scan steps (MCL)"() -> (w5038:u64)
                n3183 = Select(t=w5017, s=w5020, f=w5018) -> (s? t:f=w5019:u64)
                n3184 = Boolean To (0,1)(Boolean=w5020) -> (0, 1=w5022:i16)
                n3185 = local read "Save ave N"() -> (w5051:dbl)
                n3186 = local read "Initial X"() -> (w5025:dbl)
                n3187 = local read "Initial Y"() -> (w5024:dbl)
                n3188 = To Double Precision Float(number=w5022) -> (double precision float=w5021:dbl)
                n3189 = Boolean To (0,1)(Boolean=w5046) -> (0, 1=w5045:i16)
                n3190 = To Double Precision Float(number=w5019) -> (double precision float=w5034:dbl)
                n3191 = To Double Precision Float(number=w5038) -> (double precision float=w5037:dbl)
                n3192 = To Double Precision Float(number=w5036) -> (double precision float=w5035:dbl)
                n3193 = To Double Precision Float(number=w5045) -> (double precision float=w5044:dbl)
                n3194 = Multiply(x=w5051, y=w5030) -> (x*y=w5050:dbl)
                n3195 = To Double Precision Float(number=w5015) -> (double precision float=w5029:dbl)
                n3196 = local read "N sets should be saved (MCL)"() -> (w5032:dbl)
                n3197 = Build Array(w5029, w5021, w5023, w5023, w5023) -> (w5027:dbl[])
                n3198 = Build Array(w5044, w5039, w5037, w5035, w5034, w5025, w5024) -> (w5041:dbl[])
                n3199 = Build Array(w5026, w5030, w5050, w5049, w5048, 3.0 ("t")) -> (w5043:dbl[])
                n3200 = Round Toward +Infinity(x=w5032) -> (ceil(x): smallest int >= x=w5033:dbl)
                n3201 = Build Array (concatenate)(w5043, w5042, w5027, w5041) -> (w5040:dbl[])
                n3202 = To Unsigned Long Integer(number=w5033) -> (unsigned 32bit integer=w5031:u32)
              }
            }
            n3203 = local read "Index"() -> (w4886:dbl)
            n3204 = call "Create new save file.vi"("Insert"="", "Ext"=".dat", "Index In"=w4886) -> ("Path Out"=w4845:path, "Index Out"=w4858:dbl)
            n3205 = local write "Save file name"(w4845) -> ()
            n3206 = local write "Index"(w4858) -> ()
            n3207 = local write "Save index"(w4858) -> ()
            n3208 = Array Size(array=w4869) -> (size(s)=w4870:i32)
            n3209 = Open/Create/Replace File(file path (use dialog)=w4845, operation (0:open)=T25."create", access (0:read/write)=enum16{"read/write", "read-only", "write-only"}."write-only") -> (refnum out=w4883:refnum<file>)  [unwired: 1 in, 4 out]
            n3210 = local write "Saving..."(TRUE ("Saving...")) -> ()
            n3211 = To Double Precision Float(number=w4870) -> (double precision float=w4868:dbl)
            n3212 = String Length(string="Comment (data description)") -> (length=w4866:i32)
            n3213 = To Double Precision Float(number=w4866) -> (double precision float=w4865:dbl)
            n3214 = Deny Access(7:w4883) -> (3:w4882:refnum<file>)  [unwired: 1 in, 2 out]
            n3215 = Build Array (concatenate)(w4868, w4869, w4865) -> (w4867:dbl[])
            n3216 = case "If fluorescence data to be saved" shown="True" w4856 {
              tunnel: w4845 -> [_ w4935]
              tunnel: [refnum<k0> refnum w4915] -> w4857
              frame False {
              }
              frame True {
                w4914 = 0.0
                n3217 = local read "APD Integration Time (s)"() -> (w4920:dbl)
                n3218 = local read "N APD Samp/step"() -> (w4913:dbl)
                n3219 = Path To String(path=w4935) -> (string=w4934:string)
                n3220 = String Length(string=w4934) -> (length=w4933:i32)
                n3221 = Subtract(x=w4933, y=4) -> (x-y=w4931:i32)
                n3222 = String Subset(string=w4934, length (rest)=w4931) -> (substring=w4930:string)  [unwired: 1 out]
                n3223 = Build Array(w4920, w4913, w4914, w4914, w4914, w4914, w4914, w4914) -> (w4917:dbl[])
                n3224 = Concatenate Strings(w4930, "_fl.dat" ("string")) -> (w4928:string)
                n3225 = Array Size(array=w4917) -> (size(s)=w4919:i32)
                n3226 = String To Path(string=w4928) -> (path=w4924:path)
                n3227 = Open/Create/Replace File(file path (use dialog)=w4924, operation (0:open)=T25."create", access (0:read/write)=enum16{"read/write", "read-only", "write-only"}."write-only") -> (refnum out=w4925:refnum<file>)  [unwired: 1 in, 4 out]
                n3228 = Deny Access(7:w4925) -> (3:w4921:refnum<file>)  [unwired: 1 in, 2 out]
                n3229 = To Double Precision Float(number=w4919) -> (double precision float=w4918:dbl)
                n3230 = Build Array (concatenate)(w4918, w4917) -> (w4916:dbl[])
                n3231 = Write to Binary File(file (use dialog)=w4921, data=w4916, 5:FALSE ("prepend array or string size? (T)"), 9:T24."big-endian, network order" ("byte order (0:big-endian, network order)")) -> (refnum out=w4915:refnum<file>)  [unwired: 1 in, 3 out]
              }
            }
            n3232 = case shown="True" w4843 {
              tunnel: w4845 -> [_ w4897]
              tunnel: [refnum<k0> refnum w4896] -> w4844
              frame False {
              }
              frame True {
                w4892 = 0.0 ("element")
                n3233 = Path To String(path=w4897) -> (string=w4911:string)
                n3234 = Build Array(w4892, w4892, w4892, w4892, w4892, w4892, w4892, w4892) -> (w4893:dbl[])
                n3235 = String Length(string=w4911) -> (length=w4910:i32)
                n3236 = Subtract(x=w4910, y=4) -> (x-y=w4908:i32)
                n3237 = Array Size(array=w4893) -> (size(s)=w4895:i32)
                n3238 = String Subset(string=w4911, length (rest)=w4908) -> (substring=w4907:string)  [unwired: 1 out]
                n3239 = To Double Precision Float(number=w4895) -> (double precision float=w4894:dbl)
                n3240 = Concatenate Strings(w4907, "_pos.dat" ("string")) -> (w4905:string)
                n3241 = Build Array (concatenate)(w4894, w4893) -> (w4891:dbl[])
                n3242 = String To Path(string=w4905) -> (path=w4901:path)
                n3243 = Open/Create/Replace File(file path (use dialog)=w4901, operation (0:open)=T25."create", access (0:read/write)=enum16{"read/write", "read-only", "write-only"}."write-only") -> (refnum out=w4902:refnum<file>)  [unwired: 1 in, 4 out]
                n3244 = Deny Access(7:w4902) -> (3:w4898:refnum<file>)  [unwired: 1 in, 2 out]
                n3245 = Write to Binary File(file (use dialog)=w4898, data=w4891, 5:FALSE ("prepend array or string size? (T)"), 9:T24."big-endian, network order" ("byte order (0:big-endian, network order)")) -> (refnum out=w4896:refnum<file>)  [unwired: 1 in, 3 out]
              }
            }
            n3246 = Write to Binary File(file (use dialog)=w4882, data=w4867, 5:w4863, 9:w4861) -> (refnum out=w4864:refnum<file>)  [unwired: 1 in, 3 out]
            n3247 = Write to Binary File(file (use dialog)=w4864, data="Comment (data description)", 5:w4863, 9:w4861) -> (refnum out=w4860:refnum<file>)  [unwired: 1 in, 3 out]
          }
        }
        n3248 = feedback-in #32(w4804) -> ()
        n3249 = feedback-in #33(w4830) -> ()
        n3250 = feedback-in #34(w4803) -> ()
        n3251 = feedback-in #35(w4814) -> ()
        n3252 = feedback-in #36(w4817) -> ()
        n3253 = feedback-in #37(w4829) -> ()
        n3254 = feedback-in #38(w4820) -> ()
      }
      frame #1 {
        n3255 = local read "Saving..."() -> (w5065:bool)
        n3256 = case shown="True" w5065 {
          tunnel: w5069 -> [_ w5081]
          tunnel: w5068 -> [_ w5094]
          tunnel: w5067 -> [_ w5090]
          tunnel: w5066 -> [_ w5089]
          tunnel: w5064 -> [_ w5070]
          tunnel: w5063 -> [_ w5084]
          tunnel: w5062 -> [_ w5083]
          tunnel: w5061 -> [_ w5082]
          tunnel: w5060 -> [_ w5080]
          tunnel: w5059 -> [_ w5078]
          tunnel: w5058 -> [_ w5077]
          tunnel: w5057 -> [_ w5076]
          tunnel: w5056 -> [_ w5075]
          tunnel: w5055 -> [_ w5074]
          tunnel: w5054 -> [_ w5073]
          tunnel: w5053 -> [_ w5072]
          tunnel: w5052 -> [_ w5071]
          frame False {
          }
          frame True {
            n3257 = Multiply(x=w5081, y=w5080) -> (x*y=→"Time (s)":dbl)
            n3258 = Less Or Equal?(x=w5081, y=w5070) -> (x <= y?=w5092:bool)
            n3259 = Or(x="Stop Saving", y="Abort save 2") -> (x .or. y?=w5085:bool)
            n3260 = Not(x=w5085) -> (.not. x?=w5093:bool)
            n3261 = And(x=w5092, y=w5093) -> (x .and. y?=w5091:bool)
            n3262 = case shown="True" w5091 {
              tunnel: w5094 -> [w5102 w5177]
              tunnel: [0.0 w5180] -> w5088
              tunnel: w5081 -> [_ w5178]
              tunnel: w5070 -> [_ w5179]
              tunnel: w5090 -> [_ w5174]
              tunnel: w5089 -> [_ _]
              tunnel: w5084 -> [w5100 w5167]
              tunnel: w5083 -> [w5099 w5168]
              tunnel: w5082 -> [_ w5166]
              tunnel: w5078 -> [_ w5165]
              tunnel: w5077 -> [_ w5109]
              tunnel: w5076 -> [_ w5158]
              tunnel: w5075 -> [_ w5136]
              tunnel: w5074 -> [w5096 w5118]
              tunnel: w5073 -> [w5097 w5117]
              tunnel: w5072 -> [_ w5114]
              tunnel: w5071 -> [_ w5112]
              frame False {
                w5098 = FALSE
                n3263 = Close File(refnum=w5102) -> ()  [unwired: 1 in, 2 out]
                n3264 = case shown="True" w5099 {
                  tunnel: w5100 -> [_ w5104]
                  frame False {
                  }
                  frame True {
                    n3265 = Close File(refnum=w5104) -> ()  [unwired: 1 in, 2 out]
                  }
                }
                n3266 = case shown="True" w5096 {
                  tunnel: w5097 -> [_ w5103]
                  frame False {
                  }
                  frame True {
                    n3267 = Close File(refnum=w5103) -> ()  [unwired: 1 in, 2 out]
                  }
                }
                n3268 = call <vilib>:"Beep.vi"() -> ()  [unwired: 3 in, 9 out]
                n3269 = local write "Raster Scanning..."(w5098) -> ()
                n3270 = local write "Calibrating..."(w5098) -> ()
                n3271 = property on="Abort wiggle" class="Bool (strict)"("Val(Sgnl)"=TRUE) -> ()  [unwired: 2 in, 2 out]
                n3272 = local write "Stop Saving"(w5098) -> ()
                "Saving..." <- w5098
              }
              frame True {
                n3273 = local read "Calibrating..."() -> (w5169:bool)
                n3274 = case "Write fl. data" shown="True" w5168 {
                  tunnel: w5167 -> [_ w5203]
                  tunnel: w5166 -> [_ w5202]
                  frame False {
                  }
                  frame True {
                    n3275 = Write to Binary File(file (use dialog)=w5203, data=w5202, 5:FALSE ("prepend array or string size? (T)"), 9:T24."big-endian, network order" ("byte order (0:big-endian, network order)")) -> ()  [unwired: 1 in, 4 out]
                  }
                }
                n3276 = Greater?(x="Save ave N", y=1.0) -> (0:w5172:bool)
                n3277 = Not(x=w5169) -> (.not. x?=w5171:bool)
                n3278 = And(x=w5171, y=w5172) -> (x .and. y?=w5115:bool)
                n3279 = case shown="True" w5115 {
                  tunnel: w5114 -> [w5183 w5194]
                  tunnel: [w5183 w5186] -> w5113
                  tunnel: "Save ave N" -> [_ w5187]
                  frame False {
                  }
                  frame True {
                    w5184 = 2 ("dimension size")
                    n3280 = Array Size(array=w5194) -> (size(s)=w5188:i32)
                    n3281 = Divide(x=w5188, y=w5184) -> (x/y=w5192:dbl)
                    n3282 = Reshape Array(w5194, w5192, w5184) -> (w5193:u64[][])
                    n3283 = Transpose 2D Array(2D array=w5193) -> (transposed array=w5191:u64[][])
                    n3284 = for {
                      tunnel: w5191 -> [w5196] mode=indexing
                      tunnel: [w5195] -> w5185 mode=indexing
                      tunnel: w5187 -> [w5197]
                      workers-P: _ -> [_]
                      n3285 = call "downsample 1D array - U64.vi"("Ave N"=w5197, "Array In"=w5196) -> ("Array Out"=w5195:u64[])  [unwired: 1 in]
                    }
                    n3286 = Transpose 2D Array(2D array=w5185) -> (transposed array=w5190:u64[][])
                    n3287 = Divide(x=w5188, y=w5187) -> (x/y=w5189:dbl)
                    n3288 = Reshape Array(w5190, w5189) -> (w5186:u64[])
                  }
                }
                n3289 = case shown="True" w5115 {
                  tunnel: w5174 -> [w5206 w5218]
                  tunnel: [w5206 w5210] -> w5170
                  tunnel: "Save ave N" -> [_ w5211]
                  tunnel: w5165 -> [_ w5209]
                  frame False {
                  }
                  frame True {
                    n3290 = Array Size(array=w5218) -> (size(s)=w5212:i32)
                    n3291 = Array Size(array=w5209) -> (size(s)=w5208:i32)
                    n3292 = Divide(x=w5212, y=w5208) -> (x/y=w5216:dbl)
                    n3293 = Reshape Array(w5218, w5216, w5208) -> (w5217:i16[][])
                    n3294 = Transpose 2D Array(2D array=w5217) -> (transposed array=w5215:i16[][])
                    n3295 = for {
                      tunnel: w5215 -> [w5221] mode=indexing
                      tunnel: [w5220] -> w5207 mode=indexing
                      tunnel: w5211 -> [w5219]
                      workers-P: _ -> [_]
                      n3296 = call "downsample 1D array - I16.vi"("Ave N"=w5219, "Array In"=w5221) -> ("Array Out"=w5220:i16[])  [unwired: 1 out]
                    }
                    n3297 = Transpose 2D Array(2D array=w5207) -> (transposed array=w5214:i16[][])
                    n3298 = Divide(x=w5212, y=w5211) -> (x/y=w5213:dbl)
                    n3299 = Reshape Array(w5214, w5213) -> (w5210:i16[])
                  }
                }
                n3300 = Index Array(array=w5136, index=1) -> (element=w5139:waveform(dbl))
                n3301 = Index Array(array=w5136, index=0) -> (element=w5141:waveform(dbl))
                n3302 = Unbundle By Name(w5139) -> ("Y"=w5143:dbl[])
                n3303 = Unbundle By Name(w5141) -> ("Y"=w5151:dbl[])
                n3304 = case "Write trap pos. data" shown="True" w5118 {
                  tunnel: w5117 -> [_ w5199]
                  tunnel: w5113 -> [_ w5198]
                  frame False {
                  }
                  frame True {
                    n3305 = Write to Binary File(file (use dialog)=w5199, data=w5198, 5:FALSE ("prepend array or string size? (T)"), 9:T24."big-endian, network order" ("byte order (0:big-endian, network order)")) -> ()  [unwired: 1 in, 4 out]
                  }
                }
                n3306 = Write to Binary File(file (use dialog)=w5177, data=w5170, 5:FALSE ("prepend array or string size? (T)"), 9:T24."big-endian, network order" ("byte order (0:big-endian, network order)")) -> ()  [unwired: 1 in, 4 out]
                n3307 = feedback #39(w5143) -> (w5145:dbl[])
                n3308 = Build Array (concatenate)(w5145, w5143) -> (w5144:dbl[])
                n3309 = Select(t=w5143, s=w5109, f=w5144) -> (s? t:f=w5129:dbl[])
                n3310 = feedback-in #39(w5129) -> ()
                n3311 = feedback #40(w5151) -> (w5164:dbl[])
                n3312 = Build Array (concatenate)(w5164, w5151) -> (w5163:dbl[])
                n3313 = Select(t=w5151, s=w5109, f=w5163) -> (s? t:f=w5138:dbl[])
                n3314 = feedback-in #40(w5138) -> ()
                n3315 = Divide(x=w5178, y=w5179) -> (x/y=w5181:dbl)
                n3316 = Multiply(x=w5181, y=100.0) -> (x*y=w5180:dbl)
                n3317 = Build Array(w5138, w5129) -> (→"Saved APD":dbl[][])
                n3318 = Array Size(array=w5138) -> (size(s)=w5156:i32)
                n3319 = Unbundle By Name(w5158) -> ("Y"=w5162:dbl[])
                n3320 = Subtract(x=w5156, y="N pts to average") -> (x-y=w5132:i32)
                n3321 = Multiply(x="N pts to average", y=u16 2) -> (x*y=w5133:u16)
                n3322 = Subtract(x=w5156, y=w5133) -> (x-y=w5131:i32)
                n3323 = feedback #41(w5162) -> (w5161:dbl[])
                n3324 = Build Array (concatenate)(w5161, w5162) -> (w5160:dbl[])
                n3325 = Select(t=w5162, s=w5109, f=w5160) -> (s? t:f=w5159:dbl[])
                "Trap Delta Graph" <- w5159
                n3326 = feedback-in #41(w5159) -> ()
                n3327 = Array Subset(array=w5138, index=w5132, length="N pts to average") -> (w5155:dbl[])
                n3328 = Array Subset(array=w5138, index=w5131, length="N pts to average") -> (w5154:dbl[])
                n3329 = Array Subset(array=w5129, index=w5132, length="N pts to average") -> (w5135:dbl[])
                n3330 = Array Subset(array=w5129, index=w5131, length="N pts to average") -> (w5134:dbl[])
                n3331 = Index Array(array=w5112, index=0) -> (element=w5110:waveform(dbl))
                n3332 = call-poly <vilib>:"Mean.vi"("X"=w5155) -> ("mean"=w5153:dbl)  [unwired: 1 out]
                n3333 = call-poly <vilib>:"Mean.vi"("X"=w5135) -> ("mean"=w5128:dbl)  [unwired: 1 out]
                n3334 = call-poly <vilib>:"Mean.vi"("X"=w5154) -> ("mean"=w5152:dbl)  [unwired: 1 out]
                n3335 = call-poly <vilib>:"Mean.vi"("X"=w5134) -> ("mean"=w5127:dbl)  [unwired: 1 out]
                n3336 = Unbundle By Name(w5110) -> ("Y"=w5107:dbl[])
                n3337 = Subtract(x=w5128, y=w5127) -> (x-y=w5119:dbl)
                "Delta Fl. 2" <- w5119
